vi "Sensor Type to String.vi"(11 "Sensor Type":T1) -> (3 "Sensor String":string)   [LabVIEW 2019]
uses:
  Messages/Typedefs/Sensor Types.ctl
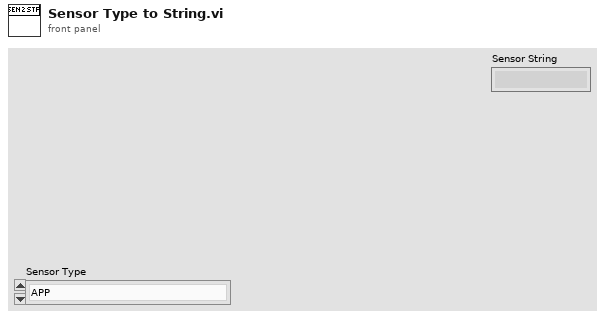
[diagram p1: front panel]
types:
  T1 = typedef "Sensor Types.ctl" = enum16{"APP", "TURBIDITY", "PH"}
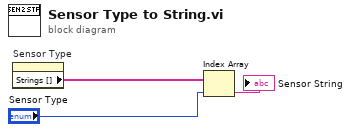
[diagram p0: block diagram]
diagram:
  n1 = property on="Sensor Type" class="Enum (strict)"() -> ("Strings []"=w3:string[])  [unwired: 2 in, 2 out]
  n2 = Index Array(array=w3, index="Sensor Type") -> (element=→"Sensor String":string)
